vi "_Parse IEM Result.vi"(8 "error in (no error)":errorcluster, 10 "Input String":string, 11 "VISA resource name":refnum<visa-resource-name>) -> (0 "error out":errorcluster, 1 "Result":T1 {"Carrier Leakage" format="%^.3e"; "IQ Image" format="%^.3e"; "General" format="%^.3e"; "Out Of Tolerance" format="%^.3e"}, 2 "Reliability":i32, 3 "VISA resource name out":refnum<visa-resource-name>)   [LabVIEW 2020, in "Rohde&Schwarz CMXP NR FR2 Measurement.lvlib"]
uses:
  <instrlib>/Rohde&Schwarz CMXP NR FR2 Measurement/Rohde&Schwarz CMXP NR FR2 Measurement.lvlib
  <instrlib>/Rohde&Schwarz CMXP NR FR2 Measurement/Private/rsidr_core.llb/rsidr_core.lvlib
panel:
  out "Reliability 2":i32
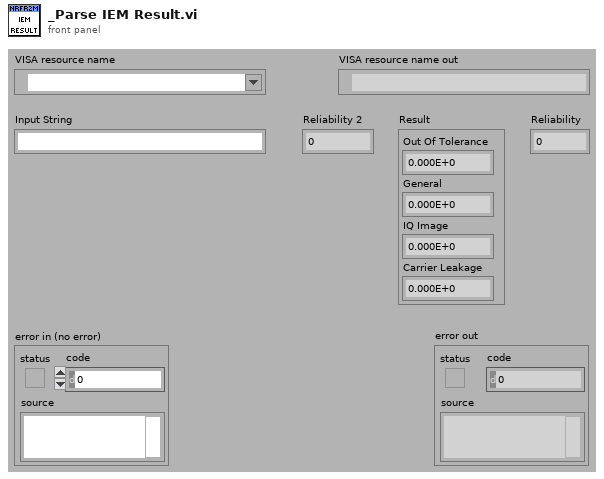
[diagram p1: front panel]
types:
  T1 = cluster{"Out Of Tolerance":dbl, "General":dbl, "IQ Image":dbl, "Carrier Leakage":dbl}
  T2 = cluster{"double array out[0]":dbl, "double array out[1]":dbl, "double array out[2]":dbl, "double array out[3]":dbl}
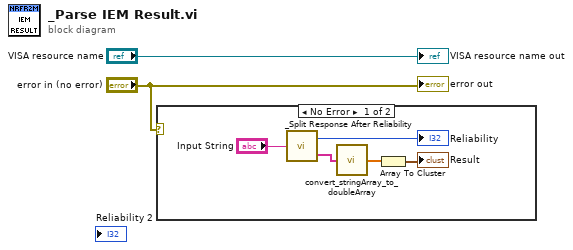
[diagram p0: block diagram]
diagram:
  n1 = case shown="No Error" "error in (no error)" {
    frame No Error {
      n2 = call <instrlib>:"_Split Response After Reliability.vi"("Input String"="Input String") -> ("Response out"=w5:string[], "Reliability out"=→"Reliability":i32)
      n3 = call <instrlib>:"convert_stringArray_to_doubleArray.vi"("string array in"=w5) -> ("double array out"=w3:dbl[])  [unwired: 4 in]
      n4 = Array To Cluster(array=w3) -> (cluster=→"Result":T2)
    }
    frame Error {
    }
  }
  "VISA resource name out" <- "VISA resource name"
  "error out" <- "error in (no error)"
